vi "changeControlState.vi"(6 "라벨명(str)":string[](array[string]), 8 "error in":errorcluster caption="에러 입력", 9 "라벨명":string[](array[string])=["Jog Control Velocity Profile", "Position Control Veclocity Profile"], 10 "기능":enum16{"LOAD", "SAVE"}(ring), 11 "VI 참조":refnum<vi>) -> (0 "error out":errorcluster caption="에러 출력")   [LabVIEW 2018]
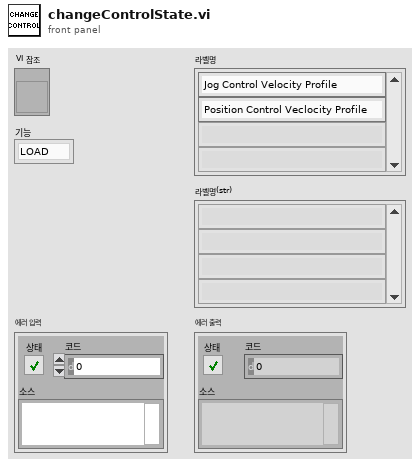
[diagram p1: front panel]
types:
  T1 = enum16{"open", "replace", "create", "open or create", "replace or create", "replace or create with confirmation"}
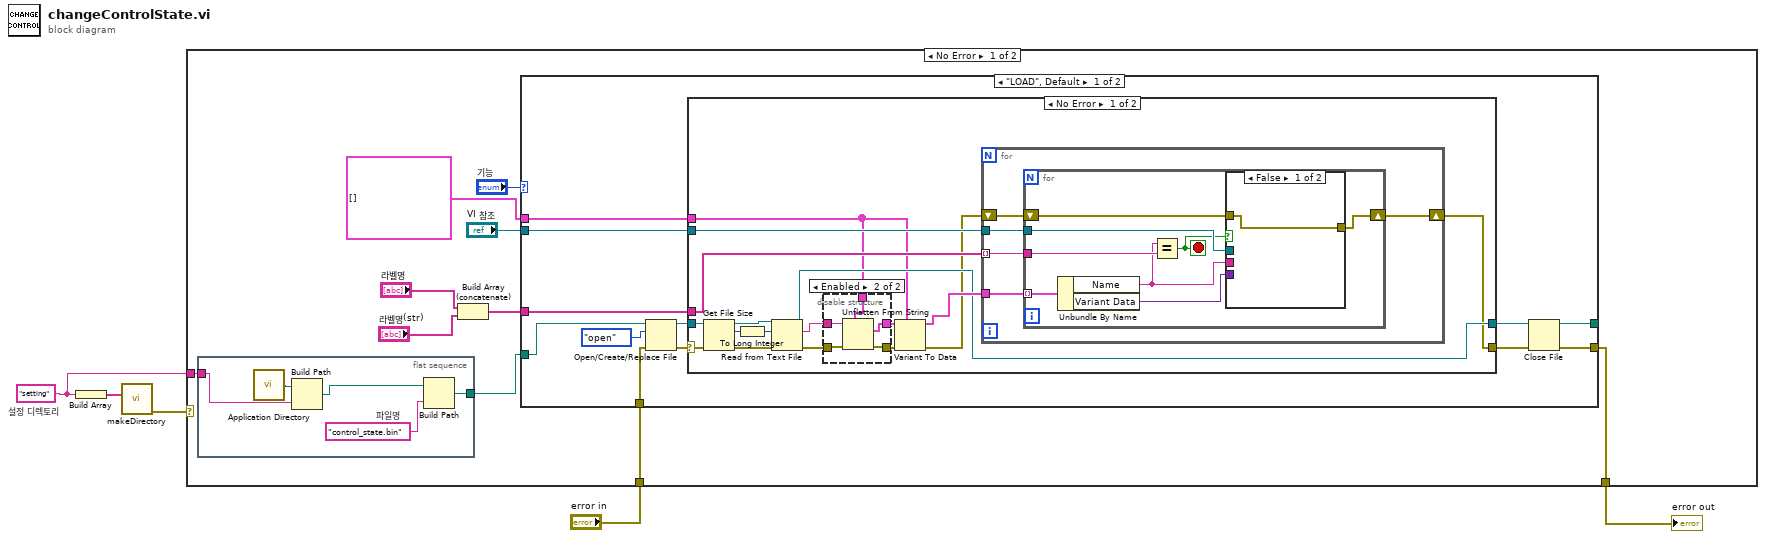
[diagram p0: block diagram]
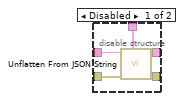
[diagram p2: hidden frame]
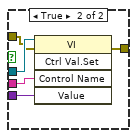
[diagram p3: hidden frame]
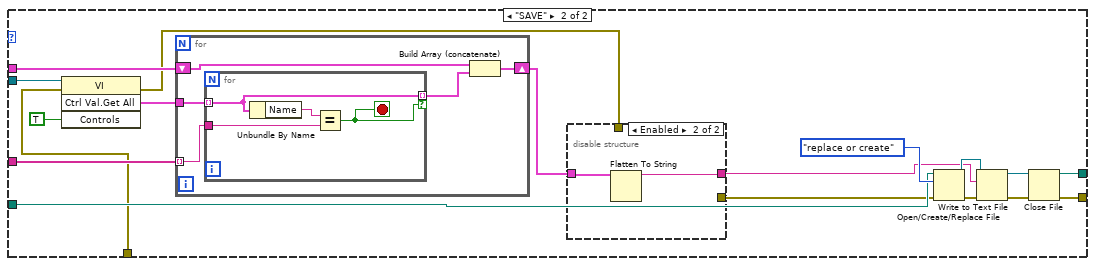
[diagram p5: hidden frame]
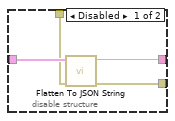
[diagram p6: hidden frame]
diagram:
  w1 = "setting"  # 설정 디렉토리
  n1 = Build Array(w1) -> (w5:string[])
  n2 = call "makeDirectory.vi"("설정 디렉토리"=w5) -> ("error out"=w4:errorcluster)  [unwired: 10 in]
  n3 = case shown="No Error" w4 {
    tunnel: "error in" -> [w8 w114]
    tunnel: [w7 w114] -> w2
    tunnel: w1 -> [w6 _]
    frame No Error {
      n4 = flat-sequence {
        tunnel: [w20] -> w13
        tunnel: w6 -> [w17]
        frame #0 {
          w19 = "control_state.bin"  # 파일명
          n5 = call <vilib>:"Application Directory.vi"() -> ("Application Directory"=w18:path)
          n6 = Build Path(base path=w18, name or relative path=w17) -> (appended path=w16:path)
          n7 = Build Path(base path=w16, name or relative path=w19) -> (appended path=w20:path)
        }
      }
      n8 = Build Array (concatenate)("라벨명", "라벨명(str)") -> (w9:string[])
      n9 = case shown="\"LOAD\", Default" "기능" {
        tunnel: w9 -> [w28 w87]
        tunnel: [w22 w82] -> _
        tunnel: [w21 w81] -> w7
        tunnel: w13 -> [w31 w95]
        tunnel: cluster{"Name":string, "Variant Data":variant}[] [] ("컨트롤 값:모두 얻기") -> [w30 w94]
        tunnel: "VI 참조" -> [w26 w89]
        tunnel: w8 -> [w25 w86]
        frame "LOAD", Default {
          n10 = Open/Create/Replace File(file path (use dialog)=w31, error in=w25, operation (0:open)=T1."open" ("동작(0:open)")) -> (refnum out=w29:refnum<file>, error out=w27:errorcluster)  [unwired: 3 in, 1 out]
          n11 = case shown="No Error" w27 {
            selector: w27 -> [w41 w80]
            tunnel: w30 -> [w37 _]
            tunnel: [w47 w79] -> w24
            tunnel: w29 -> [w43 w79]
            tunnel: w28 -> [w49 _]
            tunnel: [w33 w80] -> w23
            tunnel: w26 -> [w38 _]
            frame No Error {
              n12 = Get File Size(file=w43, error in=w41) -> (refnum out=w42:refnum<file>, size (in bytes)=w44:i64, 0:w40:errorcluster)
              n13 = To Long Integer(number=w44) -> (32bit integer=w39:i32)
              n14 = Read from Text File(file (use dialog)=w42, count=w39, error in=w40) -> (refnum out=w47:refnum<file>, text=w45:string, error out=w46:errorcluster)  [unwired: 1 in, 1 out]
              n15 = disable-structure shown="Enabled" {
                disable-tunnel: w46 -> [w54 w58]
                disable-tunnel: w45 -> [w53 w57]
                disable-tunnel: w37 -> [w52 w56]
                disable-tunnel: [w51 w55] -> w36
                disable-tunnel: [w50 w59] -> w35
                frame Disabled {
                  n16 = call "Unflatten From JSON String.vi"("Type and Defaults"=w52, "error in (no error)"=w54, "JSON String"=w53) -> ("error out"=w50:errorcluster, "Variant"=w51:variant)  [unwired: 7 in]
                }
                frame Enabled {
                  n17 = Unflatten From String(type=w56, binary string=w57, error in (no error)=w58) -> (value=w55:cluster{"Name":string, "Variant Data":variant}[], error out=w59:errorcluster)  [unwired: 2 in, 1 out]
                }
              }
              n18 = Variant To Data(error in=w35, type=w37, Variant=w36) -> (data=w48:cluster{"Name":string, "Variant Data":variant}[], error out=w34:errorcluster)
              n19 = for {
                tunnel: w48 -> [w64]
                tunnel: w49 -> [w63] mode=indexing
                tunnel: w38 -> [w62]
                shift-right: [w60] -> w33
                shift-left: w34 -> [w61]
                n20 = for {
                  tunnel: w64 -> [w72] mode=indexing
                  tunnel: w63 -> [w71]
                  tunnel: w62 -> [w68]
                  shift-right: [w65] -> w60
                  shift-left: w61 -> [w66]
                  stop <- w67 stop-if-true
                  n21 = Unbundle By Name(w72) -> ("Name"=w70:string, "Variant Data"=w69:variant)
                  n22 = Equal?(x=w70, y=w71) -> (x = y?=w67:bool)
                  n23 = case shown="False" w67 {
                    tunnel: w70 -> [_ w78]
                    tunnel: w69 -> [_ w77]
                    tunnel: w68 -> [_ w76]
                    tunnel: w66 -> [w73 w75]
                    tunnel: [w73 w74] -> w65
                    frame False {
                    }
                    frame True {
                      n24 = invoke class="VI" method="Ctrl Val.Set"(reference=w76, error in=w75, "Control Name"=w78, "Value"=w77) -> (error out=w74:errorcluster)  [unwired: 1 in, 4 out]
                    }
                  }
                }
              }
            }
            frame Error {
            }
          }
          n25 = Close File(refnum=w24, error in=w23) -> (path=w22:path, error out=w21:errorcluster)
        }
        frame "SAVE" {
          n26 = invoke class="VI" method="Ctrl Val.Get All"(reference=w89, error in=w86, "Controls"=TRUE ("컨트롤")) -> (error out=w85:errorcluster, "Get All Control Values Variant"=w92:cluster{"Name":string, "Variant Data":variant}[])  [unwired: 1 in, 2 out]
          n27 = for {
            tunnel: w92 -> [w109]
            tunnel: w87 -> [w108] mode=indexing
            shift-right: [w107] -> w88
            shift-left: w94 -> [w106]
            n28 = for {
              tunnel: w109 -> [w110] mode=indexing
              tunnel: w108 -> [w112]
              tunnel: [w110] -> w105 mode=indexing if=w111
              stop <- w111 stop-if-true
              n29 = Unbundle By Name(w110) -> ("Name"=w113:string)
              n30 = Equal?(x=w113, y=w112) -> (x = y?=w111:bool)
            }
            n31 = Build Array (concatenate)(w106, w105) -> (w107:cluster{"Name":string, "Variant Data":variant}[])
          }
          n32 = disable-structure shown="Enabled" {
            disable-tunnel: [w102 w103] -> w91
            disable-tunnel: [w101 _] -> w90
            disable-tunnel: w88 -> [w100 w104]
            disable-tunnel: w85 -> [w99 _]
            frame Disabled {
              n33 = call "Flatten To JSON String.vi"("error in (no error)"=w99, "Variant"=w100) -> ("error out"=w101:errorcluster, "JSON String"=w102:string)  [unwired: 8 in]
            }
            frame Enabled {
              n34 = Flatten To String(anything=w104) -> (data string=w103:string)  [unwired: 3 in, 2 out]
            }
          }
          n35 = Open/Create/Replace File(file path (use dialog)=w95, error in=w90, operation (0:open)=T1."replace or create" ("동작(0:open)")) -> (refnum out=w97:refnum<file>, error out=w98:errorcluster)  [unwired: 3 in, 1 out]
          n36 = Write to Text File(file (use dialog)=w97, text=w91, error in=w98) -> (refnum out=w84:refnum<file>, error out=w83:errorcluster)  [unwired: 1 in, 1 out]
          n37 = Close File(refnum=w84, error in=w83) -> (path=w82:path, error out=w81:errorcluster)
        }
      }
    }
    frame Error {
    }
  }
  "error out" <- w2
